vi "Main Page.vi"(8 "error in (no error)":errorcluster, 11 "Node Ptr":T3 format="%.0x") -> (0 "error out":errorcluster)   [LabVIEW 2014, in "SLSC configuration System Explorer.lvlib"]
uses:
  SLSC configuration System Explorer.lvlib
  <vilib>/NI Veristand/Custom Device API/Custom Device Item Ref.ctl
  Shared/Type Defs/RIO Device Address.ctl
  Type Defs/Valid.ctl
  Shared/Constants.vi
  <vilib>/NI Veristand/Custom Device API/Get Item Property (U16).vi
  <vilib>/NI Veristand/Custom Device API/Get Item Property (U32).vi
  <vilib>/NI Veristand/Custom Device API/Get Item Property (Dependent File).vi
  <vilib>/NI Veristand/Custom Device API/Get Item Property (String).vi
  <vilib>/NI Veristand/Custom Device API/Set Item Property (U16).vi
  <vilib>/NI Veristand/Custom Device API/Set Item Property (U32).vi
  <vilib>/NI Veristand/Custom Device API/Set Item Property (String).vi
  <vilib>/NI Veristand/Custom Device API/Custom Device API.lvlib
  Shared/SLSC configuration Shared.lvlib
  <vilib>/NI Veristand/Custom Device Tools/Custom Device Utility Library/Custom Device Utility Library.lvlib
panel:
  out "Valid?":T1
  out "SLSC SPI Version":string
  out "Custom Device Version":string
  in  "Header 5":cluster{"Section Name":string}={"Section Name"="Slot Configuration"}
  out "Slot Configuration":string[][](table)
  out "SPI Clock Frequency (Hz)":dbl
  in  "Sample Rate (S/s)":u32 min=1 max=40000000
  in  "FPGA Load Delay (s)":u8
  in  "SPI Divide Value":u8 min=1
  in  "Header 4":cluster{"Section Name":string}={"Section Name"="SPI Configuration"}
  in  "Header 3":cluster{"Section Name":string}={"Section Name"="FPGA Configuration"}
  in  "RIO Device Address":T2="RIO0"
  in  "Path":path
  in  "Header":cluster{"Section Name":string}={"Section Name"="SLSC Custom Device Settings"}
  in  "Name":string
  # "120 MHz"
  # "___________________________________"
  # "="
  # "("
  # "+ 1) x 2"
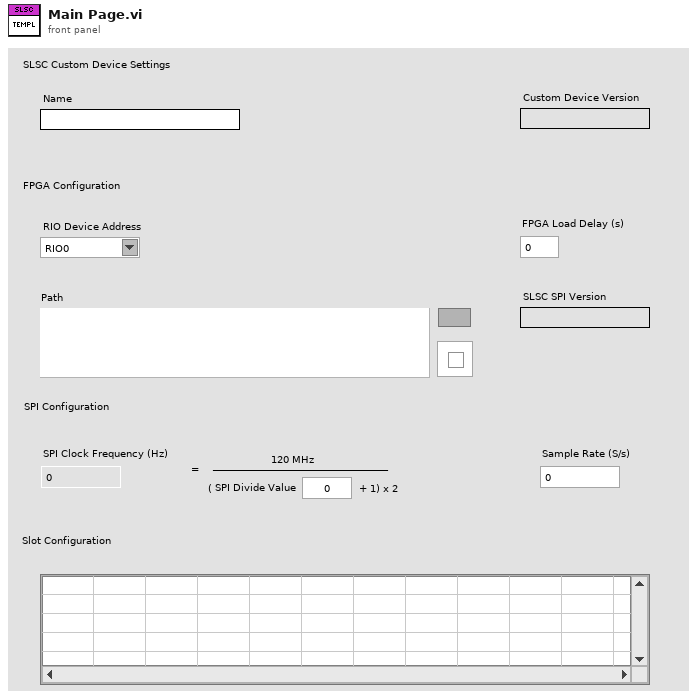
[diagram p1: front panel]
types:
  T1 = typedef "SLSC configuration System Explorer.lvlib/Valid.ctl" = bool
  T2 = typedef "SLSC configuration System Explorer.lvlib/RIO Device Address.ctl" = string
  T3 = typedef "Custom Device API.lvlib/Custom Device Item Ref.ctl" = u64
  T4 = typedef "Custom Device API.lvlib/Custom Device Item Info.ctl" = cluster{"Name":string, "Is Channel":bool, "GUID":string, "Is Waveform":bool}
  T5 = typedef "SLSC configuration System Explorer.lvlib/SLSC Bitfile Info.ctl" = cluster{"FPGA Settings":string, "FIFO Name":string, "Max # of Racks":u8, "UEGO Simulation Names":string[]}
  T6 = typedef "SLSC configuration Shared.lvlib/Card Position.ctl" = cluster{"Rack #":u8, "Slot #":T7}
  T7 = typedef "SLSC configuration Shared.lvlib/Slot #.ctl" = u8
  T8 = typedef "Custom Device API.lvlib/Custom Device Commands.ctl" = enum16{"Default", "Item renamed", "Shutdown", "Dynamic button pressed"}
  T9 = typedef "LVPoint32TypeDef.ctl" = cluster{"Horizontal":i32, "Vertical":i32}
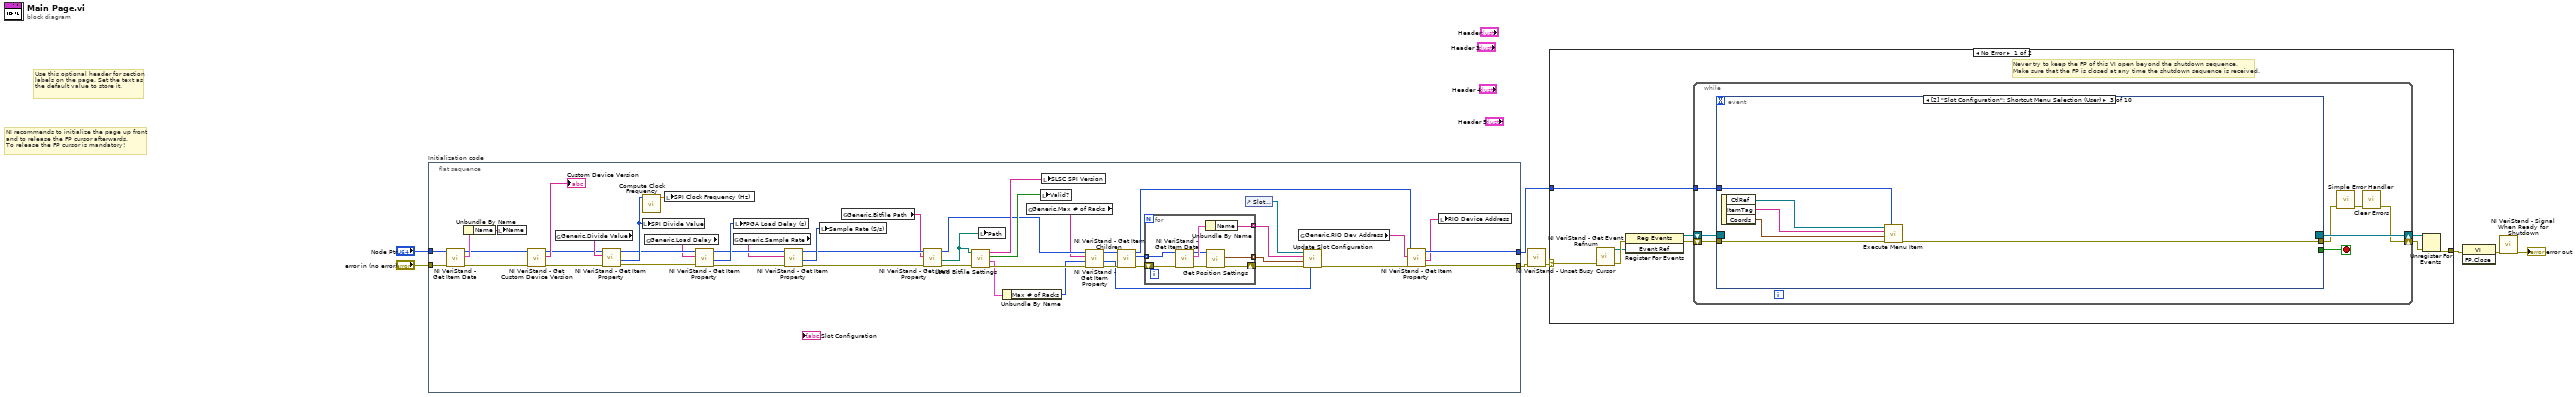
[diagram p0: block diagram]
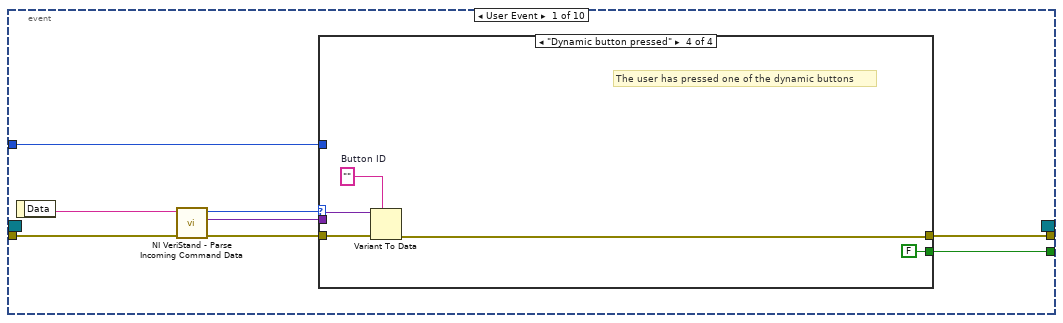
[diagram p2: hidden frame]
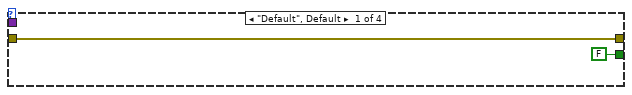
[diagram p3: hidden frame]
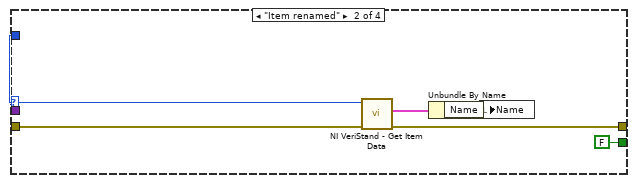
[diagram p4: hidden frame]
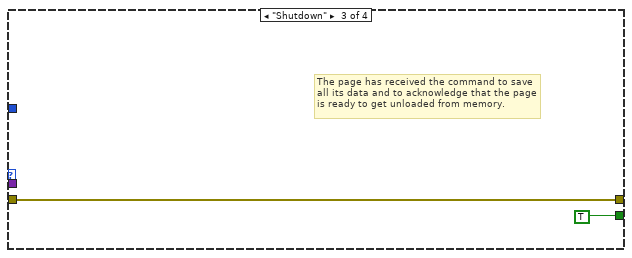
[diagram p5: hidden frame]
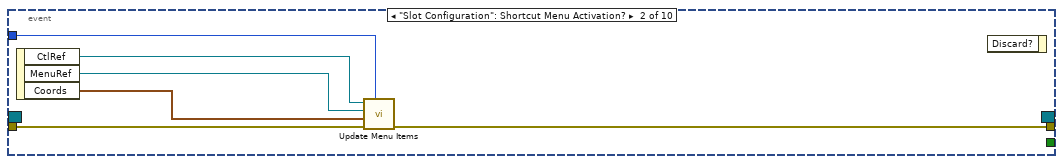
[diagram p6: hidden frame]
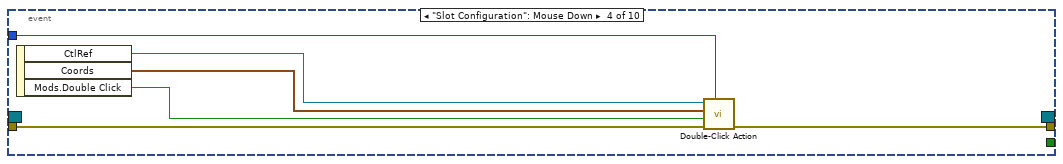
[diagram p7: hidden frame]
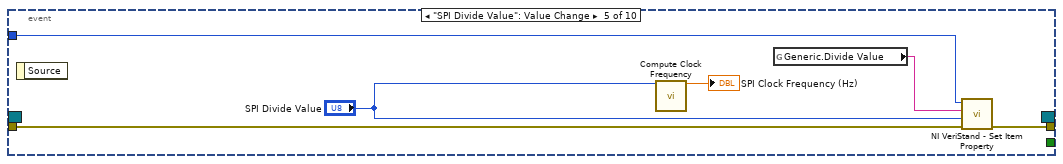
[diagram p8: hidden frame]
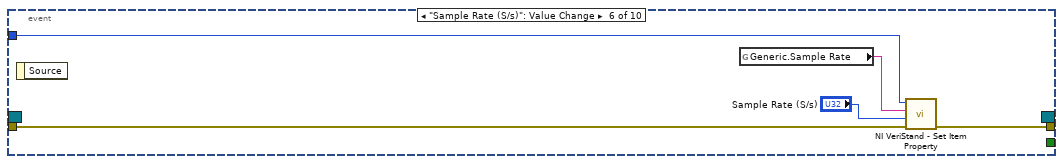
[diagram p9: hidden frame]
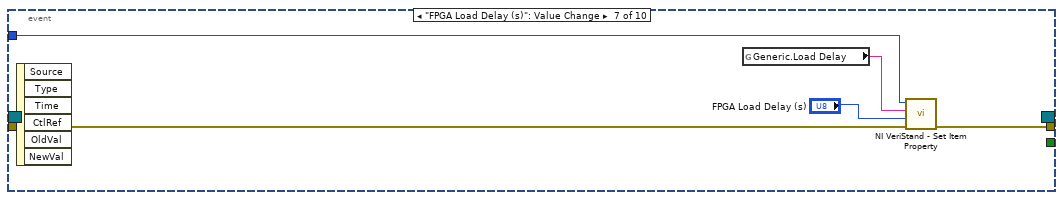
[diagram p10: hidden frame]
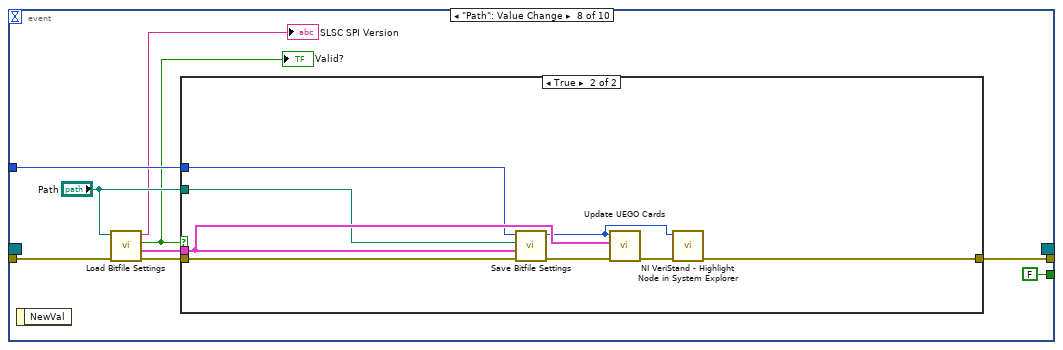
[diagram p11: hidden frame]
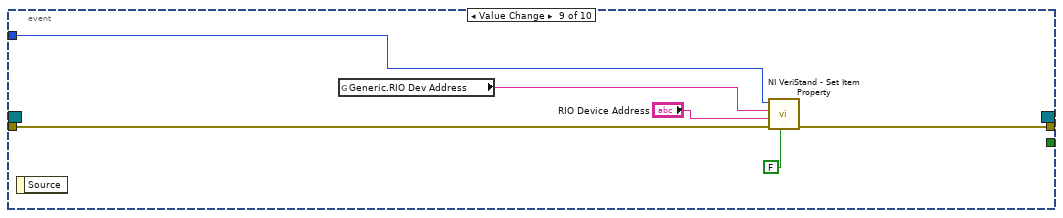
[diagram p13: hidden frame]
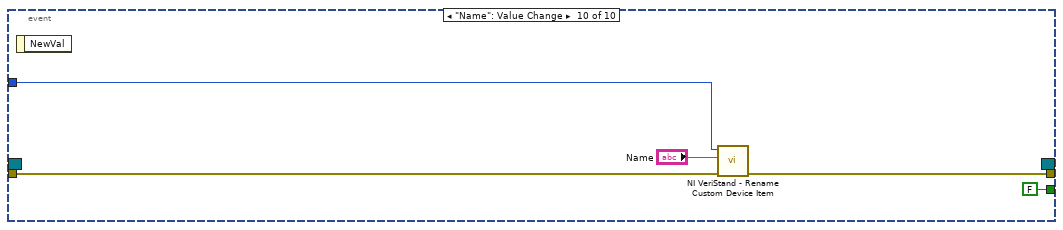
[diagram p14: hidden frame]
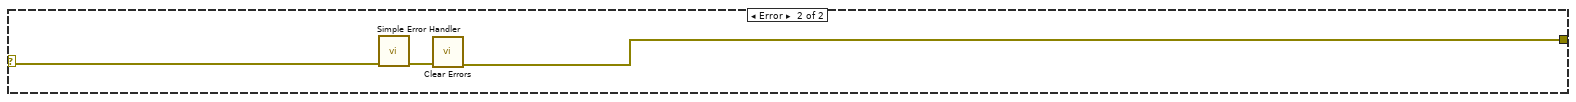
[diagram p15: hidden frame]
diagram:
  # "Use this optional header for section labels on the page. Set the text as the default value to store it."
  # "NI recommends to initialize the page up front\nand to release the FP cursor afterwards.\nTo release the FP cursor is mandatory!"
  n1 = flat-sequence "Initialization code" {
    tunnel: "error in (no error)" -> [w34]
    tunnel: "Node Ptr" -> [w35]
    tunnel: [w38] -> w4
    tunnel: [w37] -> w1
    frame #0 {
      n2 = call <vilib>:"NI VeriStand - Get Item Data.vi"("error in (no error)"=w34, "Item Ref in"=w35) -> ("error out"=w26:errorcluster, "Item Info"=w55:T4, "Item Ref out"=w27:T3)  [unwired: 7 out]
      n3 = Unbundle By Name(w55) -> ("Name"=w54:string)
      n4 = local write "Name"(w54) -> ()
      n5 = call <vilib>:"NI VeriStand - Get Custom Device Version.vi"("error in (no error)"=w26, "Device Ref in"=w27) -> ("error out"=w19:errorcluster, "Value"=→"Custom Device Version":string, "Device Ref out"=w20:T3)  [unwired: 7 in]
      n6 = global read "Constants.vi" "Generic.Divide Value"() -> (w53:string)
      n7 = call-poly <vilib>:"NI VeriStand - Get Item Property.vi"("error in (no error)"=w19, "Property Name"=w53, "Item Ref in"=w20) -> ("error out"=w50:errorcluster, "Value"=w52:u16, "Item Ref out"=w49:T3)  [unwired: 5 in, 1 out]
      n8 = call "Compute Clock Frequency.vi"("SPI Divide Value"=w52) -> ("SPI Clock Frequency (Hz)"=w51:dbl)  [unwired: 10 in]
      n9 = local write "SPI Divide Value"(w52) -> ()
      n10 = global read "Constants.vi" "Generic.Load Delay"() -> (w48:string)
      n11 = local write "SPI Clock Frequency (Hz)"(w51) -> ()
      n12 = call-poly <vilib>:"NI VeriStand - Get Item Property.vi"("error in (no error)"=w50, "Property Name"=w48, "Item Ref in"=w49) -> ("error out"=w46:errorcluster, "Value"=w47:u16, "Item Ref out"=w45:T3)  [unwired: 5 in, 1 out]
      n13 = global read "Constants.vi" "Generic.Sample Rate"() -> (w44:string)
      n14 = local write "FPGA Load Delay (s)"(w47) -> ()
      n15 = call-poly <vilib>:"NI VeriStand - Get Item Property.vi"("error in (no error)"=w46, "Property Name"=w44, "Item Ref in"=w45) -> ("error out"=w42:errorcluster, "Value"=w43:u32, "Item Ref out"=w41:T3)  [unwired: 5 in, 1 out]
      n16 = local write "Sample Rate (S/s)"(w43) -> ()
      n17 = global read "Constants.vi" "Generic.Bitfile Path"() -> (w40:string)
      n18 = call-poly <vilib>:"NI VeriStand - Get Item Property.vi"("error in (no error)"=w42, "Property Name"=w40, "Item Ref in"=w41) -> ("error out"=w24:errorcluster, "Path"=w23:path, "Item Ref out"=w18:T3)  [unwired: 4 in, 2 out]
      n19 = call "Load Bitfile Settings.vi"("error in (no error)"=w24, "bitfile path"=w23) -> ("error out"=w16:errorcluster, "Bitfile Info"=w15:T5, "Valid?"=w21:bool, "SLSC version string"=w22:string)  [unwired: 6 in]
      n20 = local write "Path"(w23) -> ()
      n21 = Unbundle By Name(w15) -> ("Max # of Racks"=w14:u8)
      n22 = global read "Constants.vi" "Generic.Max # of Racks"() -> (w17:string)
      n23 = local write "Valid?"(w21) -> ()
      n24 = local write "SLSC SPI Version"(w22) -> ()
      n25 = call-poly <vilib>:"NI VeriStand - Get Item Property.vi"("error in (no error)"=w16, "Default Value"=w14, "Property Name"=w17, "Item Ref in"=w18) -> ("error out"=w13:errorcluster, "Value"=w9:u32, "Item Ref out"=w12:T3)  [unwired: 4 in, 1 out]
      n26 = call <vilib>:"NI VeriStand - Get Item Children.vi"("error in (no error)"=w13, "Item Ref in"=w12) -> ("error out"=w32:errorcluster, "Child Refs"=w33:T3[], "Item Ref out"=w10:T3)  [unwired: 6 in, 1 out]
      n27 = for {
        tunnel: w33 -> [w63] mode=indexing
        shift-right: [w57] -> w31
        shift-left: w32 -> [w62]
        tunnel: [w60] -> w29 mode=indexing
        tunnel: [w56] -> w28 mode=indexing
        n28 = call <vilib>:"NI VeriStand - Get Item Data.vi"("error in (no error)"=w62, "Item Ref in"=w63) -> ("error out"=w59:errorcluster, "Item Info"=w61:T4, "Item Ref out"=w58:T3)  [unwired: 7 out]
        n29 = Unbundle By Name(w61) -> ("Name"=w60:string)
        n30 = call "Get Position Settings.vi"("error in (no error)"=w59, "Item Ref in"=w58) -> ("error out"=w57:errorcluster, "Card Position"=w56:T6)  [unwired: 7 in, 1 out]
      }
      n31 = control-ref of="Slot Configuration"() -> (w30:refnum<vi>)
      n32 = global read "Constants.vi" "Generic.RIO Dev Address"() -> (w39:string)
      n33 = call "Update Slot Configuration.vi"("Max # of Racks"=w9, "error in (no error)"=w31, "Card Position"=w28, "Card Name"=w29, "Slot Configuration in"=w30) -> ("error out"=w11:errorcluster)  [unwired: 5 in, 1 out]
      n34 = call-poly <vilib>:"NI VeriStand - Get Item Property.vi"("error in (no error)"=w11, "Property Name"=w39, "Item Ref in"=w10) -> ("error out"=w38:errorcluster, "Value"=w36:string, "Item Ref out"=w37:T3)  [unwired: 5 in, 1 out]
      n35 = local write "RIO Device Address"(w36) -> ()
    }
  }
  n36 = call <vilib>:"NI VeriStand - Unset Busy Cursor.vi"("error in (no error)"=w4) -> ("error out"=w3:errorcluster)  [unwired: 10 out]
  n37 = case shown="No Error" w3 {
    selector: w3 -> [w64 w169]
    tunnel: [w69 w167] -> w8
    tunnel: w1 -> [w65 _]
    frame No Error {
      # "Never try to keep the FP of this VI open beyond the shutdown sequence.\nMake sure that the FP is closed at any time the shutdown sequence is received."
      n38 = call <vilib>:"NI VeriStand - Get Event Refnum.vi"("error in (no error)"=w64) -> ("error out"=w72:errorcluster, "Event Ref"=w68:refnum<user-event>)  [unwired: 9 out]
      n39 = register-events(error in=w72, w68) -> (reference out=w66:refnum<event-registration>, error out=w67:errorcluster)  [unwired: 1 in]
      n40 = while {
        tunnel: w65 -> [w76]
        shift-right: [w73] -> w70
        shift-left: w67 -> [w79]
        shift-right: [w80] -> w71
        shift-left: w66 -> [w78]
        stop <- w77 stop-if-true
        n41 = event shown="[2] \"Slot Configuration\": Shortcut Menu Selection (User)" {
          selector: w78 -> [_ _ _ _ _ _ _ _ _ _]
          dyn-events: [_ _ _ _ _ _ _ _ _ _] -> w80
          timeout: _ -> [_ _ _ _ _ _ _ _ _ _]
          tunnel: w79 -> [w88 w107 w115 w121 w125 w132 w137 w143 w160 w166]
          tunnel: [w84 _ _ _ _ _ _ FALSE _ FALSE] -> w77
          tunnel: [w83 w106 w110 w116 w124 w131 w136 w145 w159 w165] -> w75
          tunnel: w76 -> [w82 w104 w111 w117 w126 w130 w135 w146 w158 w164]
          event User Event {
            n42 = event-data() -> ("Data"=w87:string)  [unwired: 1 out]
            n43 = call <vilib>:"NI VeriStand - Parse Incoming Command Data.vi"("error in (no error)"=w88, "Incoming data"=w87) -> ("error out"=w86:errorcluster, "Outgoing data"=w81:variant, "Action"=w85:T8)  [unwired: 7 out]
            n44 = case shown="\"Dynamic button pressed\"" w85 {
              tunnel: w86 -> [w90 w96 w97 w103]
              tunnel: [FALSE FALSE TRUE FALSE] -> w84
              tunnel: [w90 w93 w97 w100] -> w83
              tunnel: w82 -> [_ w95 _ _]
              tunnel: w81 -> [_ _ _ w102]
              frame "Default", Default {
              }
              frame "Item renamed" {
                n45 = call <vilib>:"NI VeriStand - Get Item Data.vi"("error in (no error)"=w96, "Item Ref in"=w95) -> ("error out"=w93:errorcluster, "Item Info"=w94:T4)  [unwired: 8 out]
                n46 = Unbundle By Name(w94) -> ("Name"=w92:string)
                n47 = local write "Name"(w92) -> ()
              }
              frame "Shutdown" {
                # "The page has received the command to save all its data and to acknowledge that the page is ready to get unloaded from memory."
              }
              frame "Dynamic button pressed" {
                w101 = ""  # Button ID
                # "The user has pressed one of the dynamic buttons"
                n48 = Variant To Data(error in=w103, type=w101, Variant=w102) -> (error out=w100:errorcluster)  [unwired: 1 out]
              }
            }
          }
          event "Slot Configuration": Shortcut Menu Activation? {
            n49 = event-data() -> ("CtlRef"=w109:refnum<vi>, "MenuRef"=w105:refnum<k9>, "Coords"=w108:T9)  [unwired: 1 out]
            n50 = call "Update Menu Items.vi"("Device Ref in"=w104, "error in (no error)"=w107, "Coords"=w108, "MenuRef"=w105, "Table in"=w109) -> ("error out"=w106:errorcluster)  [unwired: 6 in]
            n51 = event-data() -> ()  [unwired: 2 in, 1 out]
          }
          event "Slot Configuration": Shortcut Menu Selection (User) {
            n52 = event-data() -> ("CtlRef"=w112:refnum<vi>, "ItemTag"=w113:string, "Coords"=w114:T9)  [unwired: 1 out]
            n53 = call "Execute Menu Item.vi"("Device Ref in"=w111, "error in (no error)"=w115, "Coords"=w114, "ItemTag"=w113, "CtlRef"=w112) -> ("error out"=w110:errorcluster)  [unwired: 6 in]
          }
          event "Slot Configuration": Mouse Down {
            n54 = event-data() -> ("CtlRef"=w118:refnum<vi>, "Coords"=w119:T9, "Mods.Double Click"=w120:bool)  [unwired: 1 out]
            n55 = call "Double-Click Action.vi"("Device Ref in"=w117, "error in (no error)"=w121, "Mods.Double Click"=w120, "Coords"=w119, "CtlRef"=w118) -> ("error out"=w116:errorcluster)  [unwired: 6 in]
          }
          event "SPI Divide Value": Value Change {
            n56 = event-data() -> ()  [unwired: 2 out]
            n57 = call "Compute Clock Frequency.vi"("SPI Divide Value"="SPI Divide Value") -> ("SPI Clock Frequency (Hz)"=→"SPI Clock Frequency (Hz)":dbl)  [unwired: 10 in]
            n58 = global read "Constants.vi" "Generic.Divide Value"() -> (w127:string)
            n59 = call-poly <vilib>:"NI VeriStand - Set Item Property.vi"("error in (no error)"=w125, "Value"="SPI Divide Value", "Property Name"=w127, "Item Ref in"=w126) -> ("error out"=w124:errorcluster)  [unwired: 5 in, 2 out]
          }
          event "Sample Rate (S/s)": Value Change {
            n60 = event-data() -> ()  [unwired: 2 out]
            n61 = global read "Constants.vi" "Generic.Sample Rate"() -> (w129:string)
            n62 = call-poly <vilib>:"NI VeriStand - Set Item Property.vi"("error in (no error)"=w132, "Value"="Sample Rate (S/s)", "Property Name"=w129, "Item Ref in"=w130) -> ("error out"=w131:errorcluster)  [unwired: 5 in, 2 out]
          }
          event "FPGA Load Delay (s)": Value Change {
            n63 = event-data() -> ()  [unwired: 7 out]
            n64 = global read "Constants.vi" "Generic.Load Delay"() -> (w134:string)
            n65 = call-poly <vilib>:"NI VeriStand - Set Item Property.vi"("error in (no error)"=w137, "Value"="FPGA Load Delay (s)", "Property Name"=w134, "Item Ref in"=w135) -> ("error out"=w136:errorcluster)  [unwired: 5 in, 2 out]
          }
          event "Path": Value Change {
            n66 = event-data() -> ()  [unwired: 2 out]
            n67 = call "Load Bitfile Settings.vi"("error in (no error)"=w143, "bitfile path"="Path") -> ("error out"=w141:errorcluster, "Bitfile Info"=w139:T5, "Valid?"=w138:bool, "SLSC version string"=→"SLSC SPI Version":string)  [unwired: 6 in]
            "Valid?" <- w138
            n68 = case shown="True" w138 {
              tunnel: w146 -> [_ w152]
              tunnel: [w147 w148] -> w145
              tunnel: "Path" -> [_ w151]
              tunnel: w141 -> [w147 w155]
              tunnel: w139 -> [_ w153]
              frame False {
              }
              frame True {
                n69 = call "Save Bitfile Settings.vi"("error in (no error)"=w155, "Bitfile Info"=w153, "Path"=w151, "Device Ref in"=w152) -> ("error out"=w154:errorcluster, "Device Ref out"=w149:T3)  [unwired: 6 in]
                n70 = call "Update UEGO Cards.vi"("error in (no error)"=w154, "Bitfile Info"=w153, "Device Ref in"=w149) -> ("error out"=w150:errorcluster)  [unwired: 8 in]
                n71 = call <vilib>:"NI VeriStand - Highlight Node in System Explorer.vi"("error in (no error)"=w150, "Item Ref in"=w149) -> ("error out"=w148:errorcluster)  [unwired: 8 in, 1 out]
              }
            }
          }
          event Value Change {
            n72 = event-data() -> ()  [unwired: 2 out]
            n73 = global read "Constants.vi" "Generic.RIO Dev Address"() -> (w161:string)
            n74 = call-poly <vilib>:"NI VeriStand - Set Item Property.vi"("Binary String (T)"=FALSE, "error in (no error)"=w160, "Value"="RIO Device Address", "Property Name"=w161, "Item Ref in"=w158) -> ("error out"=w159:errorcluster)  [unwired: 4 in, 2 out]
          }
          event "Name": Value Change {
            n75 = event-data() -> ()  [unwired: 2 out]
            n76 = call <vilib>:"NI VeriStand - Rename Custom Device Item.vi"("error in (no error)"=w166, "New Name"="Name", "Item Ref in"=w164) -> ("error out"=w165:errorcluster)  [unwired: 1 in, 7 out]
          }
        }
        n77 = call <vilib>:"Simple Error Handler.vi"("error in (no error)"=w75) -> ("error out"=w74:errorcluster)  [unwired: 1 in, 7 out]
        n78 = call <vilib>:"Clear Errors.vi"("error in (no error)"=w74) -> ("error out"=w73:errorcluster)  [unwired: 1 in, 5 out]
      }
      n79 = Unregister For Events(event registration refnum=w71, error in=w70) -> (error out=w69:errorcluster)
    }
    frame Error {
      n80 = call <vilib>:"Simple Error Handler.vi"("error in (no error)"=w169) -> ("error out"=w168:errorcluster)  [unwired: 1 in, 7 out]
      n81 = call <vilib>:"Clear Errors.vi"("error in (no error)"=w168) -> ("error out"=w167:errorcluster)  [unwired: 1 in, 5 out]
    }
  }
  n82 = invoke class="VI" method="FP.Close"(error in=w8) -> (error out=w7:errorcluster)  [unwired: 2 in, 2 out]
  n83 = call <vilib>:"NI VeriStand - Signal When Ready for Shutdown.vi"("error in (no error)"=w7) -> ("error out"=→"error out":errorcluster)  [unwired: 10 out]
